vi "ReadArray.vi"(11 "files":string) -> (3 "Files":string[](array[string]))   [LabVIEW 2020]
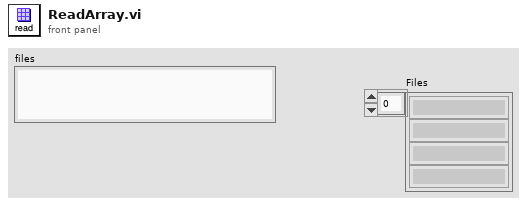
[diagram p1: front panel]
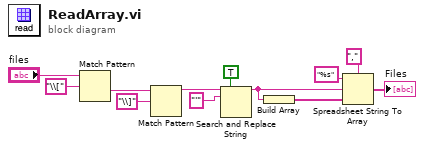
[diagram p0: block diagram]
diagram:
  n1 = Match Pattern(string="files", regular expression="\\[") -> (after substring=w2:string)  [unwired: 1 in, 3 out]
  n2 = Match Pattern(string=w2, regular expression="\\]") -> (before substring=w1:string)  [unwired: 1 in, 3 out]
  n3 = Search and Replace String(replace all?=TRUE ("replace all? (F)"), input string=w1, search string="'") -> (result string=w6:string)  [unwired: 5 in, 3 out]
  n4 = Build Array(w6) -> (w12:string[])
  n5 = Spreadsheet String To Array(delimiter (Tab)=",", format string="%s", spreadsheet string=w6, array type (2D Dbl)=w12) -> (array=→"Files":string[])
